vi "WPI_ServoGetAngle.vi"(0 "ServoDeviceRef":T1={"DeviceStatus"={"status"=FALSE, "code"=0, "source"=""}, "PWM Channel"=enum."Invalid", "DeadBand"={"Name"="", "maxPositivePwm"=0, "minPositivePwm"=0, "centerPwm"=0, "maxNegativePwm"=0, "minNegativePwm"=0, "angularRange"=0}}, 3 "error in (no error)":errorcluster) -> (7 "ServoDeviceRef":T1={"DeviceStatus"={"status"=FALSE, "code"=0, "source"=""}, "PWM Channel"=enum."Invalid", "DeadBand"={"Name"="", "maxPositivePwm"=0, "minPositivePwm"=0, "centerPwm"=0, "maxNegativePwm"=0, "minNegativePwm"=0, "angularRange"=0}}, 8 "Angle":u16, 10 "error out":errorcluster)   [LabVIEW 2017]
doc: "Returns the angle of the servo you specify.\n\nThis software is licensed. Open the labview\\readme\\WPI Robotics Library Open Source License.txt file for more information."
uses:
  <vilib>/Rock Robotics/WPI/PWM/Servo/WPI_ServoDeviceRef.ctl
  <vilib>/Rock Robotics/SystemInterfaces/DIO/FPGA_DIOPWMChannel.ctl
  <vilib>/Rock Robotics/WPI/PWM/WPI_PWMDeadband.ctl
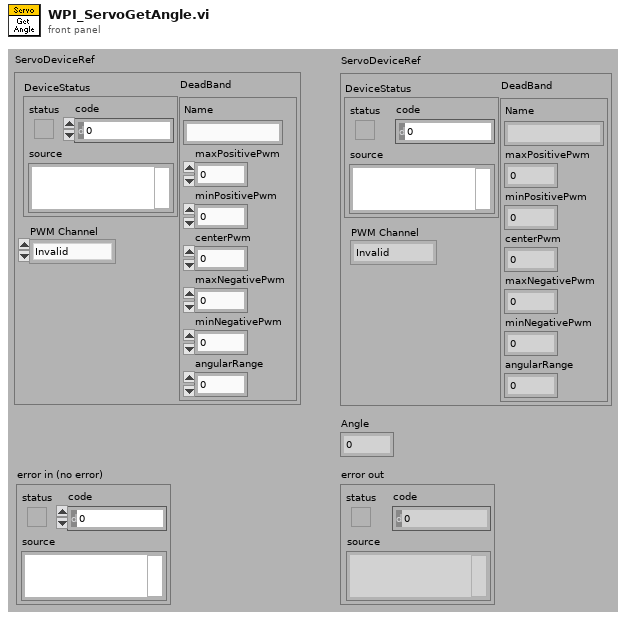
[diagram p1: front panel]
types:
  T1 = typedef "WPI_ServoDeviceRef.ctl" = cluster{"DeviceStatus":errorcluster, "PWM Channel":T2, "DeadBand":T3}
  T2 = typedef "FPGA_DIOPWMChannel.ctl" = enum8{"PWM 0", "PWM 1", "PWM 2", "PWM 3", "PWM 4", "PWM 5", "PWM 6", "PWM 7", "PWM 8", "PWM 9", "PWM MXP 0", "PWM MXP 1", "PWM MXP 2", "PWM MXP 3", "PWM MXP 4", "PWM MXP 5", "PWM MXP 6", "PWM MXP 7", "PWM MXP 8", "PWM MXP 9", "Invalid"}
  T3 = typedef "WPI_PWMDeadband.ctl" = cluster{"Name":string, "maxPositivePwm":i32, "minPositivePwm":i32, "centerPwm":i32, "maxNegativePwm":i32, "minNegativePwm":i32, "angularRange":u16}
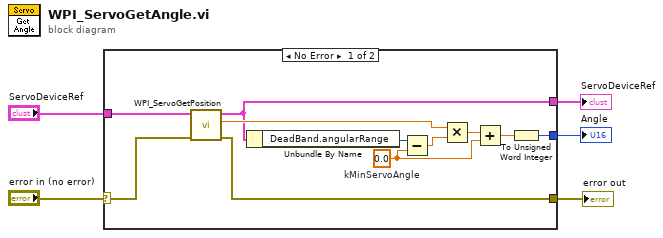
[diagram p0: block diagram]
diagram:
  n1 = case shown="No Error" "error in (no error)" {
    selector: "error in (no error)" -> [w16 w18]
    tunnel: "ServoDeviceRef" -> [w7 w17]
    tunnel: [w6 w17] -> w2
    tunnel: [w8 w18] -> w3
    tunnel: [w10 _] -> w1
    frame No Error {
      w12 = 0.0  # kMinServoAngle
      n2 = call <vilib>:"WPI_ServoGetPosition.vi"("error in (no error)"=w16, "ServoDeviceRef"=w7) -> ("error out"=w8:errorcluster, "Position"=w15:dbl, "ServoDeviceRef"=w6:T1)  [unwired: 7 out]
      n3 = Unbundle By Name(w6) -> ("DeadBand.angularRange"=w9:u16)
      n4 = Subtract(x=w9, y=w12) -> (x-y=w14:dbl)
      n5 = Multiply(x=w15, y=w14) -> (x*y=w13:dbl)
      n6 = Add(x=w13, y=w12) -> (x+y=w11:dbl)
      n7 = To Unsigned Word Integer(number=w11) -> (unsigned 16bit integer=w10:u16)
    }
    frame Error {
    }
  }
  "ServoDeviceRef" <- w2
  "Angle" <- w1
  "error out" <- w3
